vi "SubVI_Edgeelement #.vi"(8 "Error In":errorcluster, 9 "Parameter_Edge":T4={"Edge Options"={"Edge Polarity"=0, "Kernel Size"=3, "Width"=3, "Minimum Edge Strength"=10.0, "Interpolation Type"=enum."Bilinear Fixed", "Data Processing Method"=enum."Average"}, "Scan Direction"=0, "Step Size"=5, "Standard deviation"=0.0, "Auto"=FALSE} {"Edge Options"."Edge Polarity" items=["All Edges", "Rising Edges", "Falling Edges"]; "Edge Options"."Minimum Edge Strength" format="%.2f"; "Edge Options"."Width" step=2; "Edge Options"."Kernel Size" step=2; "Scan Direction" items=["Left To Right", "Right To Left", "Top To Bottom", "Bottom To Top"]}, 10 "ROI Descriptor":T1 {"Contours"."Type" items=["No Selection", "Point", "Line", "Rectangle", "Oval", "Polygon", "Free", "Annulus", "Unused2", "Unused3", "Broken Line", "Free Hand Line", "Rotated Rectangle"]}, 11 "Image In":T5) -> (0 "Error Out":errorcluster, 1 "Y Array":sgl[](array[numeric]) format="%.2g", 2 "X Array":sgl[](array[numeric]) format="%.2f", 3 "Location":cluster{"X":sgl, "Y":sgl}[](array[cluster]) {"Y" format="%.2g"; "X" format="%.2f"})   [LabVIEW 2013]
uses:
  <vilib>/vision/Image Controls.llb/IMAQ Image.ctl
  <vilib>/vision/Measure.llb/Edge Options.ctl
  <vilib>/vision/Measure.llb/Edge Polarity.ctl
  <vilib>/vision/NI_Vision_Development_Module.lvlib
panel:
  out "Image Out":T5
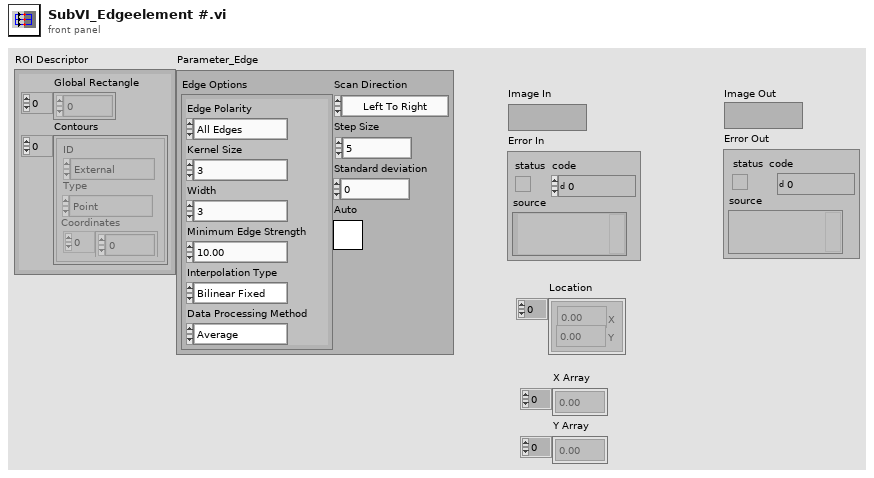
[diagram p1: front panel]
types:
  T1 = cluster{"Global Rectangle":i32[], "Contours":cluster{"ID":enum32{"External", "Internal"}, "Type":u32, "Coordinates":i32[]}[]}
  T2 = typedef "Edge Options.ctl" = cluster{"Edge Polarity":T3, "Kernel Size":u32, "Width":u32, "Minimum Edge Strength":sgl, "Interpolation Type":enum32{"Zero Order", "Bilinear", "Quadratic", "Cubic", "Bilinear Fixed"}, "Data Processing Method":enum32{"Average", "Median"}}
  T3 = typedef "Edge Polarity.ctl" = u32
  T4 = cluster{"Edge Options":T2, "Scan Direction":u16, "Step Size":u32, "Standard deviation":dbl, "Auto":bool}
  T5 = typedef "IMAQ Image.ctl" = refnum<image>
  T6 = enum16{"Get First Edge", "Get First + Last Edge", "Get All Edges", "Get Best Edge"}
  T7 = cluster{"ID":enum32{"External", "Internal"}, "Type":u32, "Coordinates":i32[]}
  T8 = typedef "ROI Descriptor" = cluster{"Global Rectangle":i32[], "Contours":cluster{"ID":enum32{"External", "Internal"}, "Type":u32, "Coordinates":i32[]}[]}
  T9 = typedef "Search Line.ctl" = cluster{"Start Point":cluster{"X":sgl, "Y":sgl}, "End Point":cluster{"X":sgl, "Y":sgl}, "Edge Info":T10[], "Edge Map":dbl[], "Calibration Valid":bool}
  T10 = typedef "Edge New.ctl" = cluster{"Location (Pixel)":cluster{"X":sgl, "Y":sgl}, "Location (Real-World)":cluster{"X":sgl, "Y":sgl}, "Distance (Pixel)":dbl, "Distance (Real-World)":dbl, "Strength":dbl, "Noise":dbl, "Rising?":bool}
  T11 = cluster{"ID":enum32{"External", "Internal"}, "Type":u32, "Coordinates":i32[]}[]
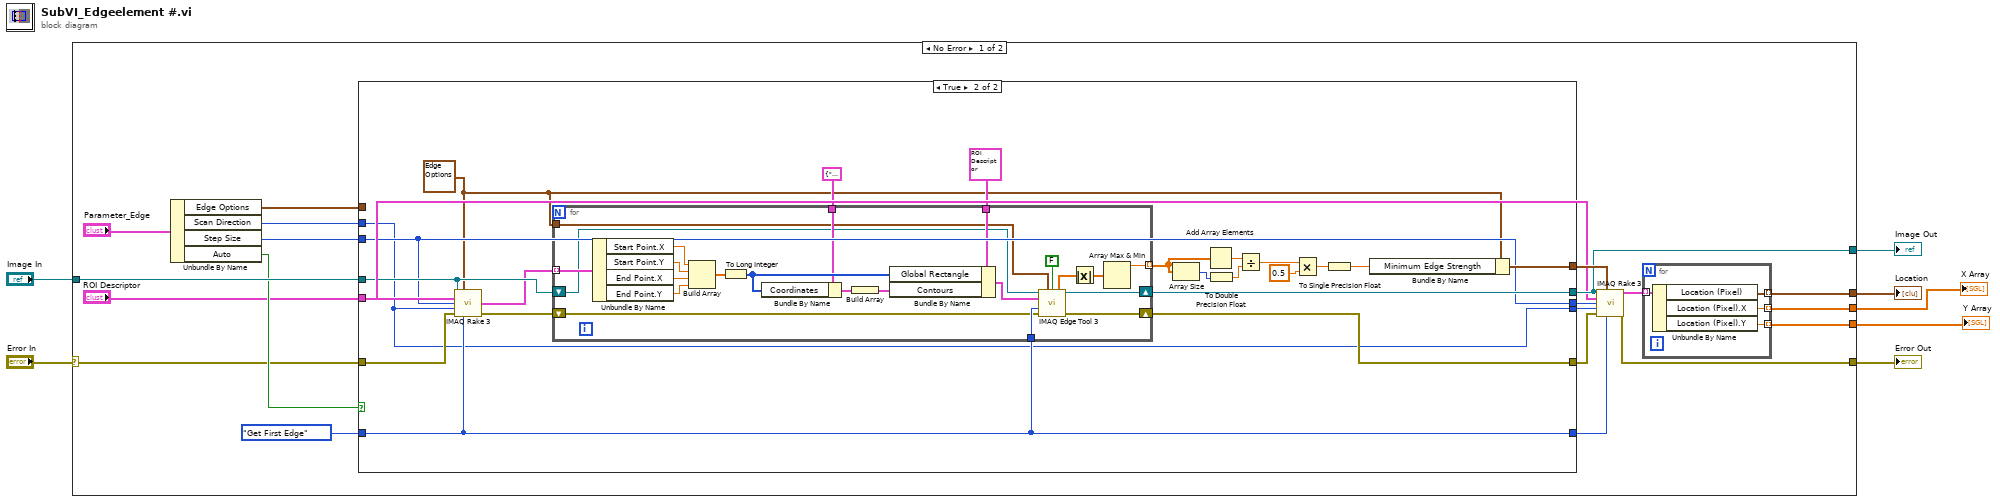
[diagram p0: block diagram]
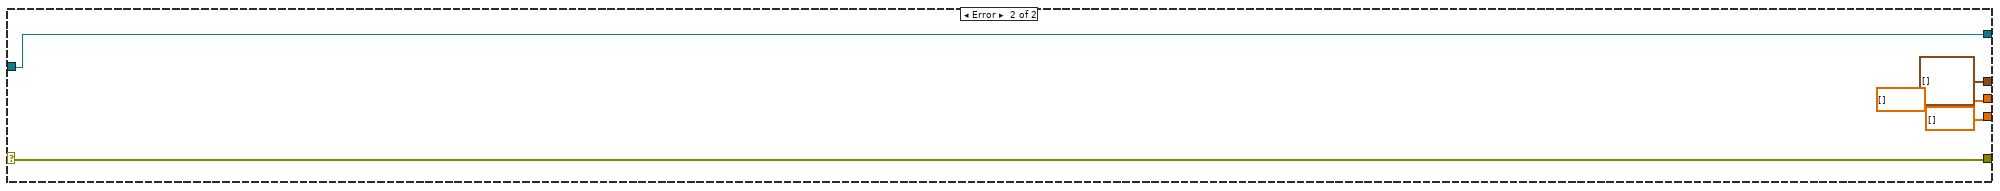
[diagram p3: hidden frame]
diagram:
  n1 = case shown="No Error" "Error In" {
    selector: "Error In" -> [w14 w85]
    tunnel: "Image In" -> [w27 w86]
    tunnel: [w13 w85] -> w5
    tunnel: [w12 w86] -> w4
    tunnel: [w11 cluster{"X":sgl, "Y":sgl}[] []] -> w3
    tunnel: [w10 sgl[] []] -> w2
    tunnel: [w9 sgl[] []] -> w1
    frame No Error {
      n2 = Unbundle By Name("Parameter_Edge") -> ("Edge Options"=w15:T2, "Scan Direction"=w16:u16, "Step Size"=w17:u32, "Auto"=w18:bool)
      n3 = case shown="True" w18 {
        tunnel: "ROI Descriptor" -> [_ w59]
        tunnel: w14 -> [w36 w58]
        tunnel: w27 -> [w37 w57]
        tunnel: [w37 w56] -> w12
        tunnel: [w32 w39] -> w26
        tunnel: [w33 w40] -> w25
        tunnel: [w34 w45] -> w24
        tunnel: [w35 w41] -> w23
        tunnel: [w36 w43] -> w22
        tunnel: T6."Get First Edge" ("Process") -> [w35 w41]
        tunnel: w15 -> [w34 _]
        tunnel: w16 -> [w32 w39]
        tunnel: w17 -> [w33 w40]
        frame False {
        }
        frame True {
          w38 = T2 {"Edge Polarity"=0, "Kernel Size"=3, "Width"=3, "Minimum Edge Strength"=10.0, "Interpolation Type"=enum."Bilinear Fixed", "Data Processing Method"=enum."Average"} ("Edge Options")
          n4 = call "IMAQ Rake 3"("Image"=w57, "Edge Options"=w38, "ROI Descriptor"=w59, "Step Size"=w40, "Scan Direction"=w39, "error in (no error)"=w58, "Process"=w41) -> ("Search Lines"=w55:T9[], "error out"=w44:errorcluster)  [unwired: 5 in, 2 out]
          n5 = for {
            tunnel: w55 -> [w81] mode=indexing
            tunnel: w41 -> [w73]
            tunnel: T8 {"Global Rectangle"=[0, 0, 0, 0], "Contours"=[{"ID"=enum."External", "Type"=2, "Coordinates"=[0, 0, 0, 0]}]} ("ROI Descriptor") -> [w71]
            tunnel: T7 {"ID"=enum."External", "Type"=2, "Coordinates"=[0, 0, 0, 0]} -> [w72]
            tunnel: w38 -> [w70]
            shift-right: [w63] -> w56
            shift-left: w57 -> [w62]
            tunnel: [w69] -> w42 mode=indexing
            shift-right: [w60] -> w43
            shift-left: w44 -> [w61]
            n6 = Unbundle By Name(w81) -> ("Start Point.X"=w80:sgl, "Start Point.Y"=w79:sgl, "End Point.X"=w78:sgl, "End Point.Y"=w77:sgl)
            n7 = Build Array(w80, w79, w78, w77) -> (w76:sgl[])
            n8 = To Long Integer(number=w76) -> (32bit integer=w74:i32[])
            n9 = Bundle By Name(cluster=w72, "Coordinates"=w74) -> (w75:T7)
            n10 = Build Array(w75) -> (w67:T11)
            n11 = Bundle By Name(cluster=w71, "Global Rectangle"=w74, "Contours"=w67) -> (w66:T8)
            n12 = call "IMAQ Edge Tool 3"("Image"=w62, "Edge Options"=w70, "Optimized Mode"=FALSE, "ROI Descriptor"=w66, "Process"=w73, "error in (no error)"=w61) -> ("Image (duplicate)"=w63:T5, "Gradient Values"=w64:dbl[], "error out"=w60:errorcluster)  [unwired: 5 in, 2 out]
            n13 = Absolute Value(x=w64) -> (abs(x)=w65:dbl[])
            n14 = Array Max & Min(array=w65) -> (max value=w69:dbl)  [unwired: 3 out]
          }
          n15 = Array Size(array=w42) -> (size(s)=w48:i32)
          n16 = Add Array Elements(numeric array=w42) -> (sum=w53:dbl)
          n17 = To Double Precision Float(number=w48) -> (double precision float=w52:dbl)
          n18 = Divide(x=w53, y=w52) -> (x/y=w51:dbl)
          n19 = Multiply(x=w51, y=0.5) -> (x*y=w47:dbl)
          n20 = To Single Precision Float(number=w47) -> (single precision float=w46:sgl)
          n21 = Bundle By Name(cluster=w38, "Minimum Edge Strength"=w46) -> (w45:T2)
        }
      }
      n22 = call "IMAQ Rake 3"("Image"=w12, "Edge Options"=w24, "ROI Descriptor"="ROI Descriptor", "Step Size"=w25, "Scan Direction"=w26, "error in (no error)"=w22, "Process"=w23) -> ("First Edges"=w21:T10[], "error out"=w13:errorcluster)  [unwired: 5 in, 2 out]
      n23 = for {
        tunnel: w21 -> [w31] mode=indexing
        tunnel: [w30] -> w11 mode=indexing
        tunnel: [w29] -> w10 mode=indexing
        tunnel: [w28] -> w9 mode=indexing
        n24 = Unbundle By Name(w31) -> ("Location (Pixel)"=w30:cluster{"X":sgl, "Y":sgl}, "Location (Pixel).X"=w29:sgl, "Location (Pixel).Y"=w28:sgl)
      }
    }
    frame Error {
    }
  }
  "Error Out" <- w5
  "Image Out" <- w4
  "Location" <- w3
  "X Array" <- w2
  "Y Array" <- w1
